vi "PhotonTrackedTarget_CreateFromPacket.vi"(9 "StartByte":i32, 11 "RawData":u8[](array[numeric])) -> (1 "NextByte":i32, 3 "TrackedTarget":T1={"Yaw"=0.0, "Pitch"=0.0, "Area"=0.0, "Skew"=0.0, "TargetCorners"=[], "BestCameraToTarget"={"TRANSLATION3D"={"X"=0.0, "Y"=0.0, "Z"=0.0}, "ROTATION3D"={"Q_quaternion"={"R"=1.0, "V"=[0.0, 0.0, 0.0]}}, "XF"=FALSE}, "FiiducialId"=0, "AltCameraToTarget"={"TRANSLATION3D"={"X"=0.0, "Y"=0.0, "Z"=0.0}, "ROTATION3D"={"Q_quaternion"={"R"=1.0, "V"=[0.0, 0.0, 0.0]}}, "XF"=FALSE}, "PoseAmbiguity"=0.0} {"AltCameraToTarget"."TRANSLATION3D"."Z" format="%14.3f"; "AltCameraToTarget"."TRANSLATION3D"."Y" format="%14.3f"; "AltCameraToTarget"."TRANSLATION3D"."X" format="%14.3f"; "BestCameraToTarget"."TRANSLATION3D"."Z" format="%14.3f"; "BestCameraToTarget"."TRANSLATION3D"."Y" format="%14.3f"; "BestCameraToTarget"."TRANSLATION3D"."X" format="%14.3f"})   [LabVIEW 2019, in "PhotonVisionLib.lvlib"]
doc: "Internal function to parse the data for each target returned by PhotonCamera_GetLatestResult.\n\nInputs:\n - RawData -- Byte array containing the data to parse.\n\nOutputs:\n - TrackedTarget -- Parsed TrackedTarget cluster."
uses:
  PhotonVisionLib.lvlib
  TypeDef/TargetCornerType.ctl
  TypeDef/PhotonTrackedTargetType.ctl
  <vilib>/Rock Robotics/WPI/ThirdParty/JAS_Junk/TrajLib/TypeDef/QUATERNION.ctl
  <vilib>/Rock Robotics/WPI/ThirdParty/JAS_Junk/TrajLib/Trajectory_Library.lvlib
  <vilib>/Rock Robotics/WPI/ThirdParty/JAS_Junk/TrajLib/TypeDef/ROTATION3D.ctl
  <vilib>/Rock Robotics/WPI/ThirdParty/JAS_Junk/TrajLib/TypeDef/TRANSLATION3D.ctl
  <vilib>/Rock Robotics/WPI/ThirdParty/JAS_Junk/TrajLib/TypeDef/TRANSFORM3D.ctl
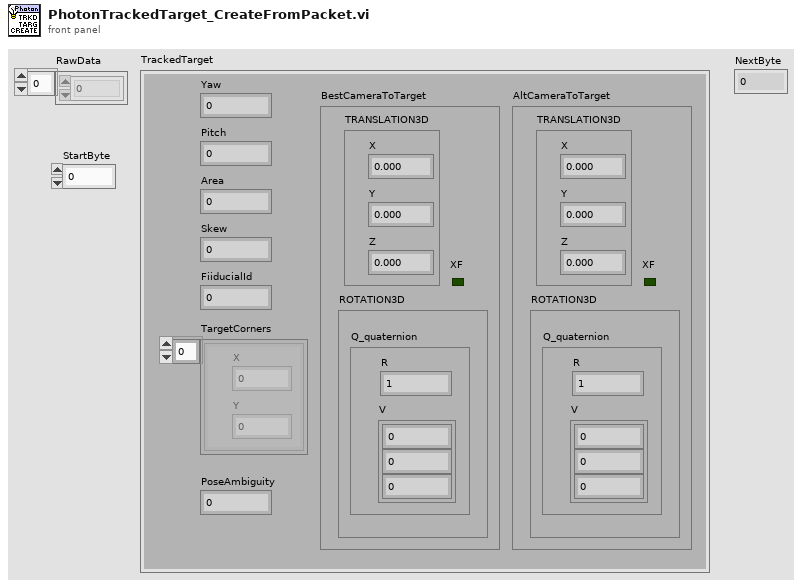
[diagram p1: front panel]
types:
  T1 = typedef "PhotonVisionLib.lvlib/PhotonTrackedTargetType.ctl" = cluster{"Yaw":dbl, "Pitch":dbl, "Area":dbl, "Skew":dbl, "TargetCorners":T2[], "BestCameraToTarget":T3, "FiiducialId":i32, "AltCameraToTarget":T3, "PoseAmbiguity":dbl}
  T2 = typedef "PhotonVisionLib.lvlib/TargetCornerType.ctl" = cluster{"X":dbl, "Y":dbl}
  T3 = typedef "Trajectory_Library.lvlib/TRANSFORM3D.ctl" = cluster{"TRANSLATION3D":T4, "ROTATION3D":T5, "XF":bool}
  T4 = typedef "Trajectory_Library.lvlib/TRANSLATION3D.ctl" = cluster{"X":dbl, "Y":dbl, "Z":dbl}
  T5 = typedef "Trajectory_Library.lvlib/ROTATION3D.ctl" = cluster{"Q_quaternion":T6}
  T6 = typedef "Trajectory_Library.lvlib/QUATERNION.ctl" = cluster{"R":dbl, "V":dbl[]}
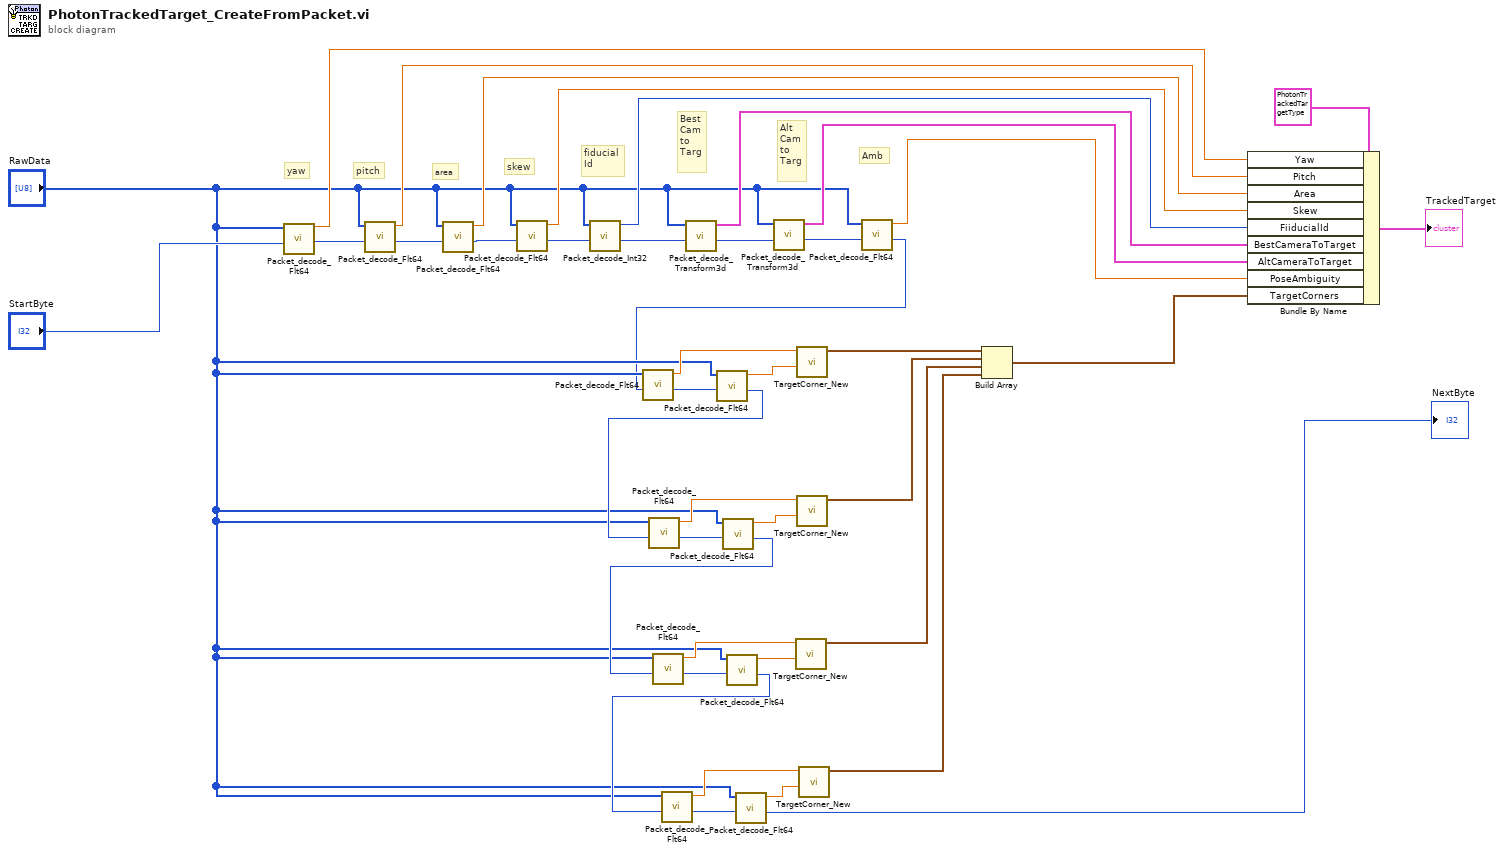
[diagram p0: block diagram]
diagram:
  # "Amb"
  # "Alt\nCam\nto\nTarg"
  # "Best\nCam\nto\nTarg"
  # "fiducial\nId"
  # "skew"
  # "area"
  # "pitch"
  # "yaw"
  n1 = call "Packet_decode_Flt64.vi"("StartByte"="StartByte", "RawData"="RawData") -> ("NextByte"=w38:i32, "Flt64_Value"=w41:dbl)  [unwired: 8 in]
  n2 = call "Packet_decode_Flt64.vi"("StartByte"=w38, "RawData"="RawData") -> ("NextByte"=w36:i32, "Flt64_Value"=w37:dbl)  [unwired: 8 in]
  n3 = call "Packet_decode_Flt64.vi"("StartByte"=w36, "RawData"="RawData") -> ("NextByte"=w25:i32, "Flt64_Value"=w31:dbl)  [unwired: 8 in]
  n4 = call "Packet_decode_Flt64.vi"("StartByte"=w25, "RawData"="RawData") -> ("NextByte"=w11:i32, "Flt64_Value"=w24:dbl)  [unwired: 8 in]
  n5 = call "Packet_decode_Int32.vi"("StartByte"=w11, "RawData"="RawData") -> ("NextByte"=w8:i32, "Int32_Value"=w10:i32)  [unwired: 8 in]
  n6 = call "Packet_decode_Transform3d.vi"("NextByte in"=w8, "RawData"="RawData") -> ("NextByte out"=w7:i32, "Transform3d"=w9:T3)  [unwired: 6 in]
  n7 = call "Packet_decode_Transform3d.vi"("NextByte in"=w7, "RawData"="RawData") -> ("NextByte out"=w4:i32, "Transform3d"=w6:T3)  [unwired: 6 in]
  n8 = call "Packet_decode_Flt64.vi"("StartByte"=w4, "RawData"="RawData") -> ("NextByte"=w3:i32, "Flt64_Value"=w1:dbl)  [unwired: 8 in]
  n9 = call "Packet_decode_Flt64.vi"("StartByte"=w3, "RawData"="RawData") -> ("NextByte"=w35:i32, "Flt64_Value"=w22:dbl)  [unwired: 8 in]
  n10 = call "Packet_decode_Flt64.vi"("StartByte"=w35, "RawData"="RawData") -> ("NextByte"=w30:i32, "Flt64_Value"=w21:dbl)  [unwired: 8 in]
  n11 = call "Packet_decode_Flt64.vi"("StartByte"=w30, "RawData"="RawData") -> ("NextByte"=w34:i32, "Flt64_Value"=w17:dbl)  [unwired: 8 in]
  n12 = call "Packet_decode_Flt64.vi"("StartByte"=w34, "RawData"="RawData") -> ("NextByte"=w29:i32, "Flt64_Value"=w16:dbl)  [unwired: 8 in]
  n13 = call "Packet_decode_Flt64.vi"("StartByte"=w29, "RawData"="RawData") -> ("NextByte"=w33:i32, "Flt64_Value"=w15:dbl)  [unwired: 8 in]
  n14 = call "Packet_decode_Flt64.vi"("StartByte"=w33, "RawData"="RawData") -> ("NextByte"=w28:i32, "Flt64_Value"=w14:dbl)  [unwired: 8 in]
  n15 = call "Packet_decode_Flt64.vi"("StartByte"=w28, "RawData"="RawData") -> ("NextByte"=w32:i32, "Flt64_Value"=w13:dbl)  [unwired: 8 in]
  n16 = call "Packet_decode_Flt64.vi"("StartByte"=w32, "RawData"="RawData") -> ("NextByte"=→"NextByte":i32, "Flt64_Value"=w12:dbl)  [unwired: 8 in]
  n17 = call "TargetCorner_New.vi"("Y"=w14, "X"=w15) -> ("TargetCorner"=w19:T2)  [unwired: 9 in]
  n18 = call "TargetCorner_New.vi"("Y"=w21, "X"=w22) -> ("TargetCorner"=w23:T2)  [unwired: 9 in]
  n19 = call "TargetCorner_New.vi"("Y"=w16, "X"=w17) -> ("TargetCorner"=w20:T2)  [unwired: 9 in]
  n20 = call "TargetCorner_New.vi"("Y"=w12, "X"=w13) -> ("TargetCorner"=w18:T2)  [unwired: 9 in]
  n21 = Build Array(w23, w20, w19, w18) -> (w2:T2[])
  n22 = Bundle By Name(cluster=T1 {"Yaw"=0.0, "Pitch"=0.0, "Area"=0.0, "Skew"=0.0, "TargetCorners"=[], "BestCameraToTarget"={"TRANSLATION3D"={"X"=0.0, "Y"=0.0, "Z"=0.0}, "ROTATION3D"={"Q_quaternion"={"R"=1.0, "V"=[0.0, 0.0, 0.0]}}, "XF"=FALSE}, "FiiducialId"=0, "AltCameraToTarget"={"TRANSLATION3D"={"X"=0.0, "Y"=0.0, "Z"=0.0}, "ROTATION3D"={"Q_quaternion"={"R"=1.0, "V"=[0.0, 0.0, 0.0]}}, "XF"=FALSE}, "PoseAmbiguity"=0.0} ("PhotonTrackedTarget"), "Yaw"=w41, "Pitch"=w37, "Area"=w31, "Skew"=w24, "FiiducialId"=w10, "BestCameraToTarget"=w9, "AltCameraToTarget"=w6, "PoseAmbiguity"=w1, "TargetCorners"=w2) -> (→"TrackedTarget":T1)
